vi "Update Project Linking.vi"(8 "error in":errorcluster, 11 "Project Path":path) -> (0 "error out":errorcluster)   [LabVIEW 2020, in "ADAS_IO_Template_MDO.lvclass"]
uses:
  ADAS_IO_Template_MDO.lvclass
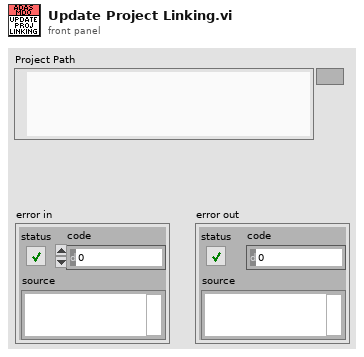
[diagram p1: front panel]
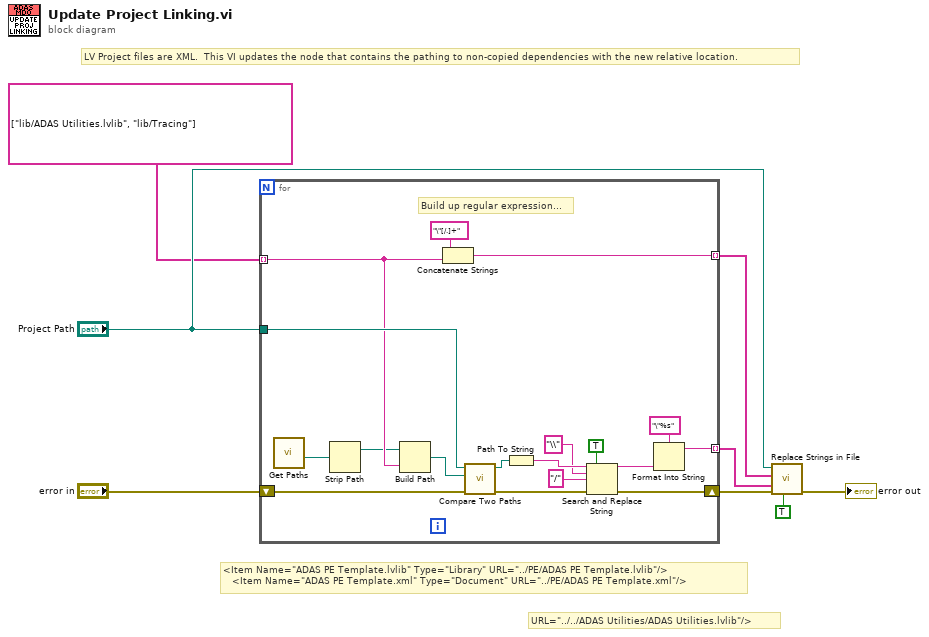
[diagram p0: block diagram]
diagram:
  # "URL=\"../../ADAS Utilities/ADAS Utilities.lvlib\"/>"
  # "<Item Name=\"ADAS PE Template.lvlib\" Type=\"Library\" URL=\"../PE/ADAS PE Template.lvlib\"/>\n\t\t\t<Item Name=\"ADAS PE Template.xml\" Type=\"Document\" URL=\"../PE/ADAS PE Template.xml\"/>"
  # "LV Project files are XML.  This VI updates the node that contains the pathing to non-copied dependencies with the new relative location."
  n1 = for {
    tunnel: string[] ["lib/ADAS Utilities.lvlib", "lib/Tracing"] -> [w12] mode=indexing
    tunnel: "Project Path" -> [w19]
    shift-right: [w17] -> w5
    shift-left: "error in" -> [w18]
    tunnel: [w16] -> w4 mode=indexing
    tunnel: [w14] -> w2 mode=indexing
    # "Build up regular expression..."
    n2 = call "Get Paths.vi"() -> ("Source Folder"=w10:path)  [unwired: 10 in, 1 out]
    n3 = Strip Path(path=w10) -> (stripped path=w9:path)  [unwired: 1 out]
    n4 = Build Path(base path=w9, name or relative path=w12) -> (appended path=w11:path)
    n5 = Concatenate Strings("\"[/.]+" ("string"), w12) -> (w14:string)
    n6 = call <vilib>:"Compare Two Paths.vi"("error in (no error)"=w18, "Path 2"=w11, "Path 1"=w19) -> ("error out"=w25:errorcluster, "Relative Path from 1 to 2"=w20:path)  [unwired: 5 in, 2 out]
    n7 = Path To String(path=w20) -> (string=w24:string)
    n8 = Search and Replace String(replace all?=TRUE ("replace all? (F)"), input string=w24, search string="\\", replace string="/" ("search string"), error in=w25) -> (result string=w13:string, error out=w17:errorcluster)  [unwired: 3 in, 2 out]
    n9 = Format Into String(format string="\"%s", w13) -> (resulting string=w16:string)  [unwired: 2 in, 1 out]
  }
  n10 = call "Replace Strings in File.vi"("Use RegEx? (F)"=TRUE, "error in"=w5, "Replace Strings"=w4, "Search Strings"=w2, "File Path"="Project Path") -> ("error out"=→"error out":errorcluster)  [unwired: 6 in]
